vi "ConnexionUDP.vi"() -> ()   [LabVIEW 2019]
uses:
  <vilib>/myRIO/Common/Instrument Driver Framework/myRIO v1.0/UART/vis/myRIO v1.0 Close UART.vi
  <vilib>/myRIO/Common/Instrument Driver Framework/Utilities/vis/FPGA Ref Manager.vi
  <vilib>/myRIO/Common/Instrument Driver Framework/myRIO v1.0/myRIO v1.0 Reset FPGA.vi
  <vilib>/myRIO/Common/Instrument Driver Framework/myRIO v1.0/IRQ/vis/myRIO v1.0 IRQ Info FGV.vi
  <vilib>/myRIO/Common/Instrument Driver Framework/myRIO v1.0/IRQ/vis/myRIO v1.0 Timer IRQ Info FGV.vi
  <vilib>/myRIO/Common/Instrument Driver Framework/myRIO v1.0/IRQ/vis/myRIO v1.0 ISR Agent.vi
  <vilib>/myRIO/Instrument Drivers/Utilities/vis/Reset Index.vi
  <vilib>/myRIO/Common/Instrument Driver Framework/myRIO v1.0/Resource Manager/vis/myRIO v1.0 Block Write Resource Manager.vi
  <vilib>/myRIO/Instrument Drivers/Utilities/Utilities.lvlib
panel:
  out "error out":errorcluster
  in  "Stop":bool
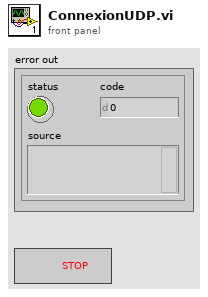
[diagram p1: front panel]
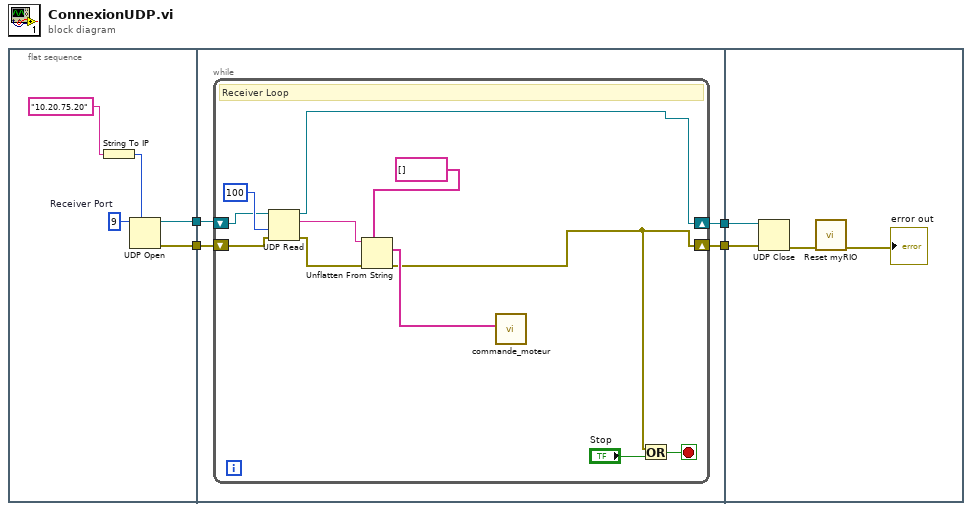
[diagram p0: block diagram]
diagram:
  n1 = flat-sequence {
    tunnel: [w8] -> w4
    tunnel: [w7] -> w3
    tunnel: [w13] -> w2
    tunnel: [w12] -> w1
    tunnel: w4 -> [w11]
    tunnel: w3 -> [w10]
    tunnel: w2 -> [w27]
    tunnel: w1 -> [w28]
    frame #0 {
      w9 = u16 9  # Receiver Port
      n2 = String To IP(1:"10.20.75.20") -> (0:w5:u32)
      n3 = UDP Open(7:w5, 11:w9) -> (port=w8:refnum<k16>, 0:w7:errorcluster)  [unwired: 3 in, 1 out]
    }
    frame #1 {
      n4 = while {
        shift-right: [w14] -> w12
        shift-left: w10 -> [w22]
        shift-right: [w19] -> w13
        shift-left: w11 -> [w20]
        stop <- w23 stop-if-true
        # "Receiver Loop"
        n5 = UDP Read(connection ID=w20, timeout ms (25000)=100, 8:w22) -> (data out=w16:string, error out=w15:errorcluster, 3:w19:refnum<k16>)  [unwired: 1 in, 2 out]
        n6 = Unflatten From String(type=string[] [], binary string=w16, error in (no error)=w15) -> (value=w18:string[], error out=w14:errorcluster)  [unwired: 2 in, 1 out]
        n7 = call "commande_moteur.vi"("liste commande"=w18) -> ()  [unwired: 11 in]
        n8 = Or(x=w14, y="Stop") -> (x .or. y?=w23:bool)
      }
    }
    frame #2 {
      n9 = UDP Close(connection ID=w27, 8:w28) -> (error out=w26:errorcluster)  [unwired: 1 out]
      n10 = call <vilib>:"Reset myRIO.vi"("error in (no error)"=w26) -> ("error out"=→"error out":errorcluster)  [unwired: 10 in]
    }
  }
